vi "Global 2.vi"() -> ()   [LabVIEW 2019]
panel:
  out "Path":path=path "E:/TSDL.csv"
  # "E:\\TSDL.csv"
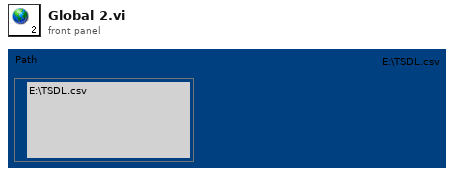
[diagram p1: front panel]
diagram:
